vi "Init.vi"(8 "error in (no error)":errorcluster, 11 "base view in":refnum<class "base view.lvclass">) -> (0 "error out":errorcluster, 3 "base view out":refnum<class "base view.lvclass">)   [LabVIEW 2022 SP3, in "base view.lvclass"]
uses:
  base view.lvclass
  Data.ctl
  Events.ctl
  base view.lvclass/base view.ctl
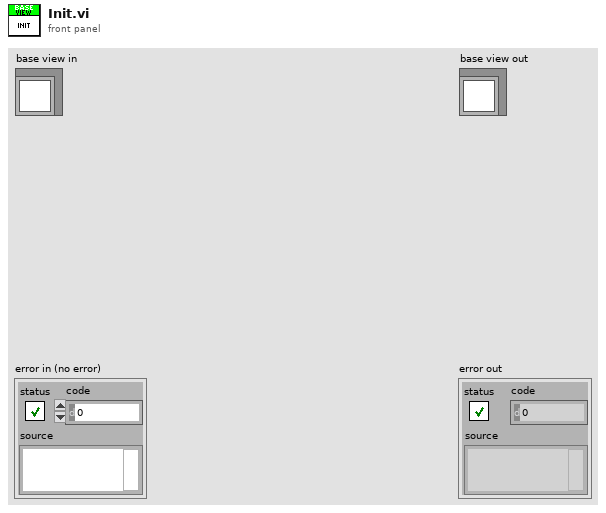
[diagram p1: front panel]
types:
  T1 = typedef "base view.lvclass/Data.ctl" = cluster{"View Refnum":refnum<vi>, "Wrapped View Refnum":refnum<vi>, "Events":T2, "event registration refnum":refnum<event-registration>}
  T2 = typedef "base view.lvclass/Events.ctl" = cluster{"Open":refnum<user-event>, "Close":refnum<user-event>, "Hide":refnum<user-event>}
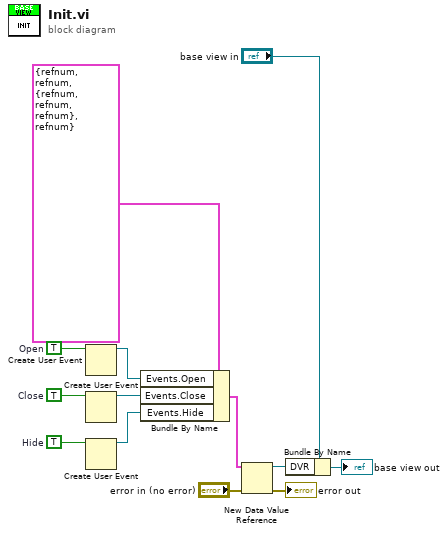
[diagram p0: block diagram]
diagram:
  w10 = TRUE  # Hide
  w11 = TRUE  # Close
  w12 = TRUE  # Open
  n1 = Create User Event(user event datatype=w12) -> (user event=w9:refnum<user-event>)  [unwired: 1 in, 1 out]
  n2 = Create User Event(user event datatype=w11) -> (user event=w8:refnum<user-event>)  [unwired: 1 in, 1 out]
  n3 = Create User Event(user event datatype=w10) -> (user event=w7:refnum<user-event>)  [unwired: 1 in, 1 out]
  n4 = Bundle By Name(cluster=T1 {"View Refnum"=refnum, "Wrapped View Refnum"=refnum, "Events"={"Open"=refnum, "Close"=refnum, "Hide"=refnum}, "event registration refnum"=refnum} ("Data"), "Events.Open"=w9, "Events.Close"=w8, "Events.Hide"=w7) -> (w5:T1)
  n5 = New Data Value Reference(data value=w5, error in="error in (no error)") -> (data value reference=w3:refnum<data-value>, error out=→"error out":errorcluster)
  n6 = Bundle By Name(cluster="base view in", "DVR"=w3) -> (→"base view out":refnum<class "base view.lvclass">)
